vi "Files Write Delimited Spreadsheet (CSL).vi"(0 "file path (dialog if empty)":path, 1 "format (%.3f)":string="%.3f", 5 "2D data":csg[][](array[numeric]), 7 "1D data":csg[](array[numeric]), 9 "append to file? (new file:F)":bool, 11 "error in (no error)":errorcluster, 12 "transpose? (no:F)":bool, 13 "delimiter (\\t)":string="\t") -> (4 "new file path (Not A Path if cancelled)":path, 15 "error out":errorcluster)   [LabVIEW 2021, in "Files.lvlib"]
doc: "Converts a 2D or 1D array of strings, signed integers, or double-precision numbers to a text string and writes the string to a new byte stream file or appends the string to an existing file. Wire data to the <B>2D data</B> input or <B>1D data</B> input to determine the polymorphic instance to use or manually select the instance.\n\nUse this VI to transpose or separate data.\n\n<B>Note</B> To format with Microsoft Excel, use ActiveX with LabVIEW or the Report Generation Toolkit for Microsoft Office."
uses:
  Files.lvlib
panel:
  in  "prompt":string="Choose file to write."
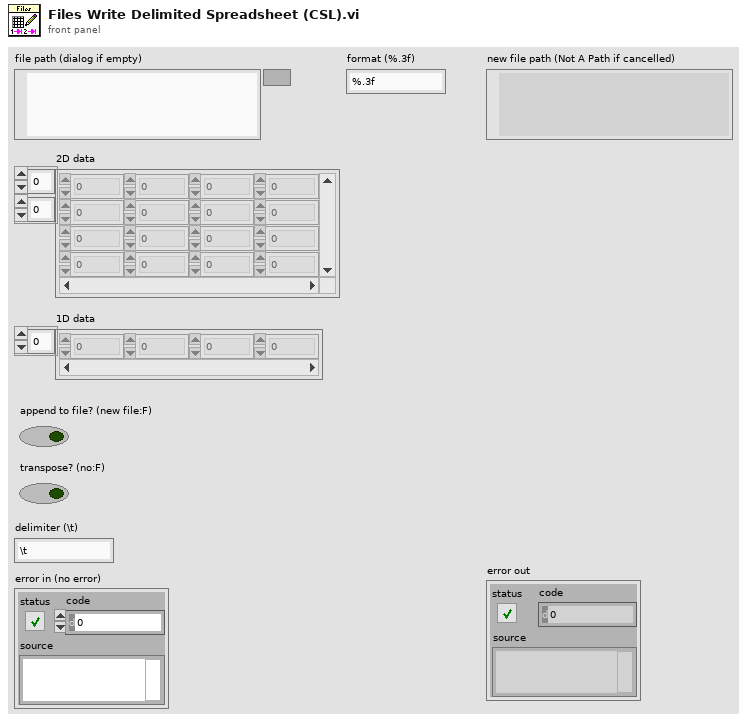
[diagram p1: front panel]
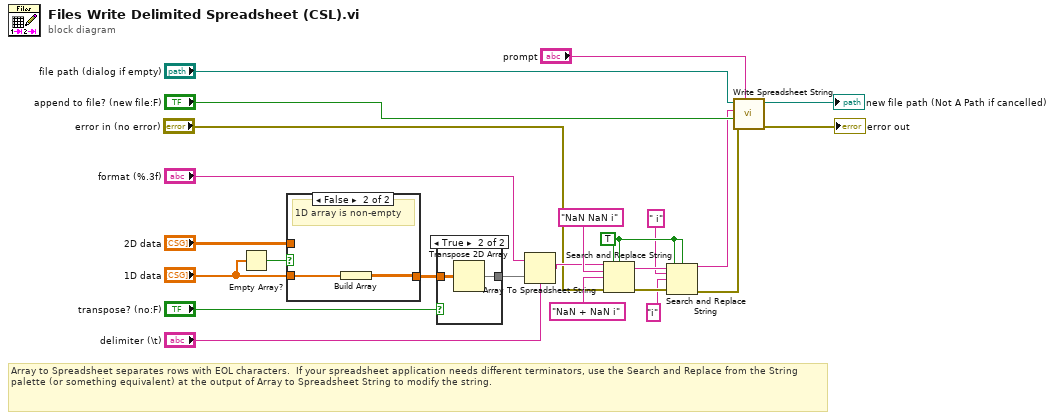
[diagram p0: block diagram]
diagram:
  w3 = TRUE ("replace all? (F)")
  # "Array to Spreadsheet separates rows with EOL characters.  If your spreadsheet application needs different terminators, use the Search and Replace from the String palette (or something equivalent) at the output of Array to Spreadsheet String to modify the string."
  n1 = Empty Array?(array="1D data") -> (empty?=w23:bool)
  n2 = case shown="False" w23 {
    tunnel: "1D data" -> [_ w27]
    tunnel: [w25 w26] -> w19
    tunnel: "2D data" -> [w25 _]
    frame True {
      # "1D array is empty"
    }
    frame False {
      # "1D array is non-empty"
      n3 = Build Array(w27) -> (w26:csg[][])
    }
  }
  n4 = case shown="True" "transpose? (no:F)" {
    tunnel: [w28 w30] -> w17
    tunnel: w19 -> [w28 w29]
    frame False {
    }
    frame True {
      n5 = Transpose 2D Array(2D array=w29) -> (transposed array=w30:csg[][])
    }
  }
  n6 = Array To Spreadsheet String(delimiter (Tab)="delimiter (\\t)", array=w17, 3:"format (%.3f)") -> (spreadsheet string=w10:string)
  n7 = Search and Replace String(replace all?=w3, case sensitive?=w3, input string=w10, search string="NaN NaN i", replace string="NaN + NaN i" ("search string"), error in="error in (no error)") -> (result string=w7:string, error out=w6:errorcluster)  [unwired: 2 in, 2 out]
  n8 = Search and Replace String(replace all?=w3, case sensitive?=w3, input string=w7, search string=" i", replace string="i" ("replace string (\"\")"), error in=w6) -> (result string=w5:string, error out=w4:errorcluster)  [unwired: 2 in, 2 out]
  n9 = call <vilib>:"Write Spreadsheet String.vi"("prompt"="prompt", "error in"=w4, "append to file? (new file:F)"="append to file? (new file:F)", "spreadsheet string"=w5, "file path (dialog if empty)"="file path (dialog if empty)") -> ("error out"=→"error out":errorcluster, "path"=→"new file path (Not A Path if cancelled)":path)  [unwired: 5 in]
